vi "Generate CSV Report combined.vi"(1 "Project":string, 2 "Serial number":string, 3 "Variant":string, 4 "Device Status":string, 5 "error in":errorcluster, 6 "First CSV":bool, 7 "Fixture number":string, 9 "Operating Mode":string) -> (19 "error out":errorcluster)   [LabVIEW 2023]
uses:
  <vilib>/Utility/file.llb/Write Delimited Spreadsheet (string).vi
panel:
  in  "Test":string
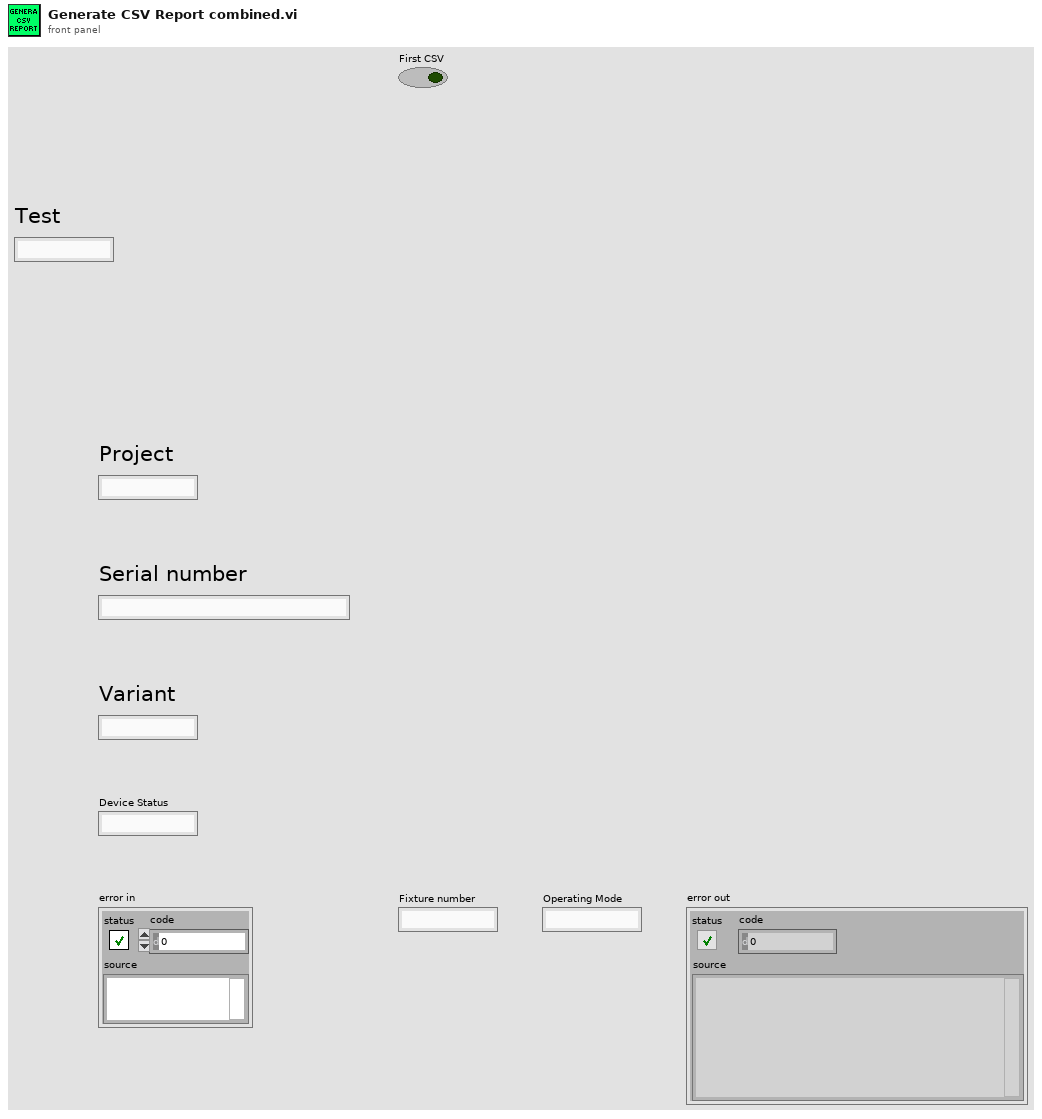
[diagram p1: front panel]
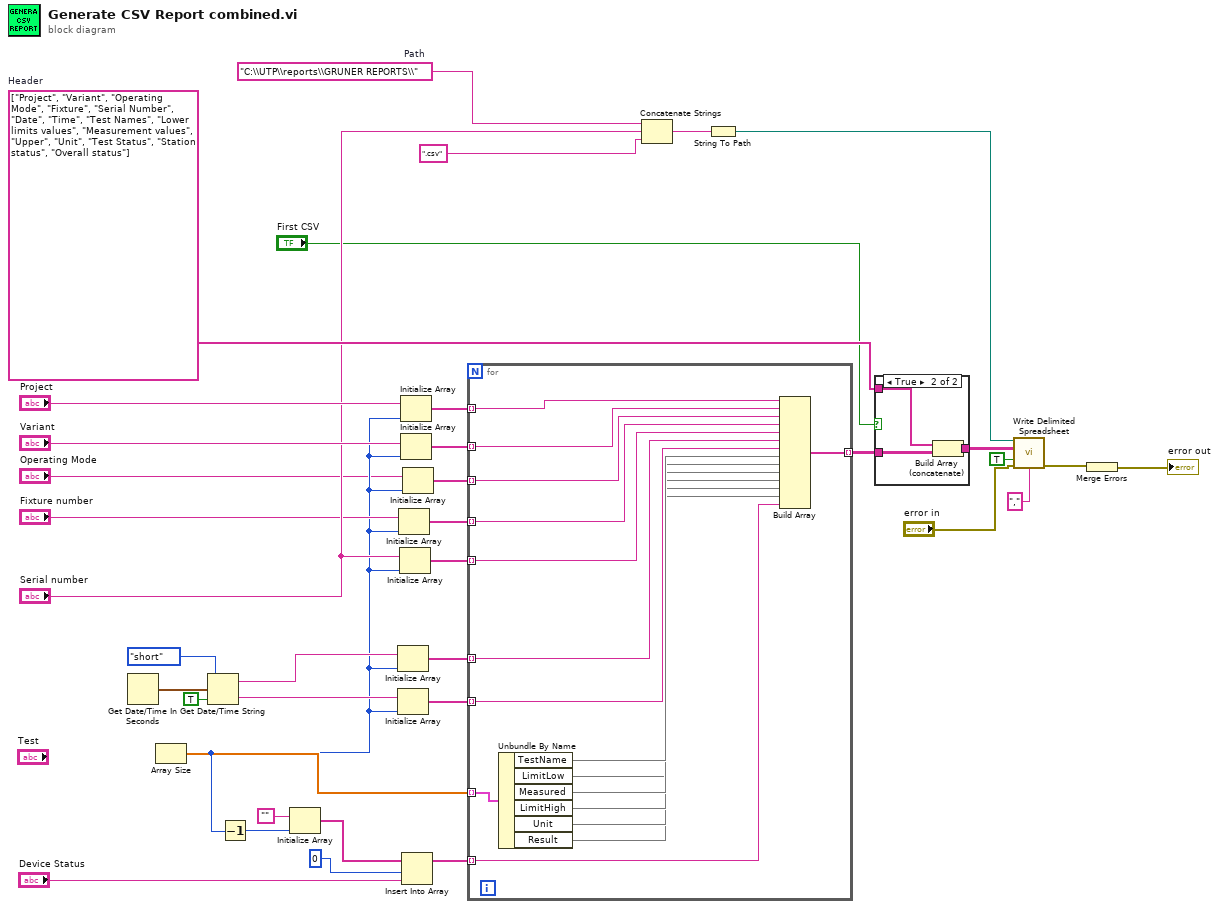
[diagram p0: block diagram]
diagram:
  w27 = "C:\\UTP\\reports\\GRUNER REPORTS\\"  # Path
  w30 = string[] ["Project", "Variant", "Operating Mode", "Fixture", "Serial Number", "Date", "Time", "Test Names", "Lower limits values", "Measurement values", "Upper", "Unit", "Test Status", "Station status", "Overall status"]  # Header
  n1 = Get Date/Time In Seconds() -> (seconds since 1Jan1904=w14:timestamp)
  n2 = Array Size() -> (array=w5:dbl[], size(s)=w3:i32)
  n3 = Get Date/Time String(date format (0)=enum16{"short", "long", "abbreviated"}."short", seconds (now)=w14, want seconds? (F)=TRUE) -> (date string=w13:string, time string=w12:string)
  n4 = Decrement(x=w3) -> (x-1=w24:i32)
  n5 = Initialize Array("", w24) -> (w20:string[])
  n6 = Initialize Array(w13, w3) -> (w35:string[])
  n7 = Initialize Array(w12, w3) -> (w34:string[])
  n8 = Initialize Array("Fixture number", w3) -> (w36:string[])
  n9 = Initialize Array("Serial number", w3) -> (w31:string[])
  n10 = Initialize Array("Project", w3) -> (w38:string[])
  n11 = Initialize Array("Variant", w3) -> (w37:string[])
  n12 = Insert Into Array(array=w20, index=0, new element="Device Status") -> (w33:string[])
  n13 = Initialize Array("Operating Mode", w3) -> (w1:string[])
  n14 = for {
    tunnel: w38 -> [w39] mode=indexing
    tunnel: w37 -> [w40] mode=indexing
    tunnel: w36 -> [w53] mode=indexing
    tunnel: w31 -> [w52] mode=indexing
    tunnel: w35 -> [w51] mode=indexing
    tunnel: w34 -> [w50] mode=indexing
    tunnel: w33 -> [w43] mode=indexing
    tunnel: [w54] -> w29 mode=indexing
    tunnel: w5 -> [w49] mode=indexing
    tunnel: w1 -> [w41] mode=indexing
    n15 = Unbundle By Name(w49) -> ("TestName"=w48, "LimitLow"=w42, "Measured"=w47, "LimitHigh"=w46, "Unit"=w45, "Result"=w44)
    n16 = Build Array(w39, w40, w41, w53, w52, w51, w50, w48, w42, w47, w46, w45, w44, w43) -> (w54:string[])
  }
  n17 = Concatenate Strings(w27, "Serial number", ".csv" ("string")) -> (w26:string)
  n18 = String To Path(string=w26) -> (path=w25:path)
  n19 = case shown="True" "First CSV" {
    tunnel: w30 -> [_ w58]
    tunnel: w29 -> [w55 w57]
    tunnel: [w55 w56] -> w28
    frame False {
    }
    frame True {
      n20 = Build Array (concatenate)(w58, w57) -> (w56:string[][])
    }
  }
  n21 = call-poly <vilib>:"Write Delimited Spreadsheet.vi"("file path (dialog if empty)"=w25, "2D data"=w28, "append to file? (new file:F)"=TRUE, "error in (no error)"="error in", "delimiter (\\t)"="," ("delimiter (\\t)")) -> ("error out"=w18:errorcluster)  [unwired: 9 in, 1 out]
  n22 = Merge Errors(w18) -> (→"error out":errorcluster)
